vi "Bring VI to Front.vi"(6 "Extra Step out of calling VI":bool, 8 "error in (no error)":errorcluster, 11 "VI in":refnum<vi>) -> (0 "error out":errorcluster)   [LabVIEW 2018]
doc: "This VI brings the calling VI to the front using a Windows library call."
uses:
  USER32.DLL
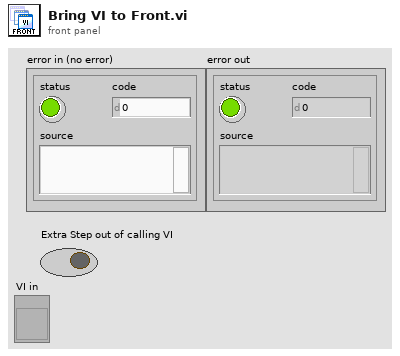
[diagram p1: front panel]
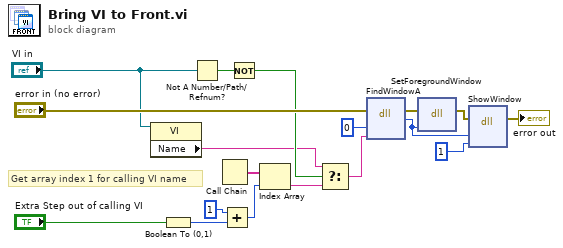
[diagram p0: block diagram]
diagram:
  # "Get array index 1 for calling VI name"
  n1 = property class="VI"(reference="VI in") -> ("Name"=w2:string)  [unwired: 1 in, 2 out]
  n2 = Boolean To (0,1)(Boolean="Extra Step out of calling VI") -> (0, 1=w8:i16)
  n3 = Not A Number/Path/Refnum?(number/path/refnum="VI in") -> (NaN/Path/Refnum?=w5:bool)
  n4 = Call Chain() -> (call chain=w14:string[])
  n5 = Add(x=1 ("index"), y=w8) -> (x+y=w10:i32)
  n6 = Not(x=w5) -> (.not. x?=w3:bool)
  n7 = Index Array(array=w14, index=w10) -> (element=w1:string)
  n8 = Select(t=w2, s=w3, f=w1) -> (s? t:f=w6:string)
  n9 = dll-call lib="user32.dll" fn="FindWindowA"(error in="error in (no error)", "arg1"=0, "arg2"=w6) -> (error out=w16:errorcluster, "return type"=w17:i32)  [unwired: 3 in, 2 out]
  n10 = dll-call lib="USER32.DLL" fn="SetForegroundWindow"(error in=w16, "arg1"=w17) -> (error out=w15:errorcluster)  [unwired: 3 in, 2 out]
  n11 = dll-call lib="user32.dll" fn="ShowWindow"(error in=w15, "arg1"=w17, "arg2"=1) -> (error out=→"error out":errorcluster)  [unwired: 4 in, 2 out]
